vi "PressureSensorModel.vi"(10 "inputSignal(V)":dbl) -> (2 "Pressure(bar)":dbl)   [LabVIEW 2020]
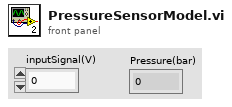
[diagram p1: front panel]
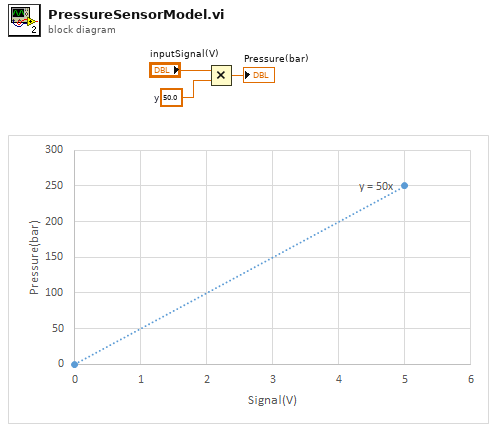
[diagram p0: block diagram]
diagram:
  w2 = 50.0  # y
  n1 = Multiply(x="inputSignal(V)", y=w2) -> (x*y=→"Pressure(bar)":dbl)
